vi "SVT Human Vibration Weighting Filter (Fixed Rates).vi"   [LabVIEW 2017, in "SoundVib_HumanVibration.lvlib"]
doc: "Applies the selected human vibration weighting to a scaled signal expressed in engineering units. This VI complies with ISO 8041:2005 (E), JIS B 7760:2004, and JISB 7761:2004 standards. Each instance of this VI maintains its own state; use the N Channel instance of this VI to process an array of channels. This VI operates on time-continuous data; it resets on a discontinuity. Wire data to the <B>scaled signal [EU]</B> input to determine the polymorphic instance to use or manually select the instance."
uses:
  <vilib>/addons/Sound and Vibration/svt_Weighting/SoundVib_HumanVibration.lvlib
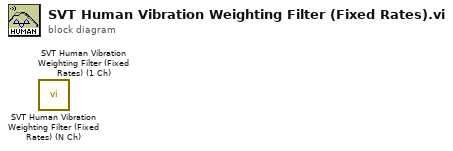
[diagram p0: block diagram]
diagram:
  n1 = call <vilib>:"SVT Human Vibration Weighting Filter (Fixed Rates) (N Ch).vi"() -> ()  [unwired: 10 in, 2 out]
  n2 = call <vilib>:"SVT Human Vibration Weighting Filter (Fixed Rates) (1 Ch).vi"() -> ()  [unwired: 10 in, 2 out]
